vi "Knob.vi"(8 "error in":errorcluster, 11 "Gen Refnum":refnum<vi>) -> (0 "error out":errorcluster, 3 "Knob out":refnum<class "Knob.lvclass">)   [LabVIEW 2014, in "Raspberry Pi Compatible Compiler for LabVIEW.lvlib" / "Knob.lvclass"]
uses:
  Knob.lvclass
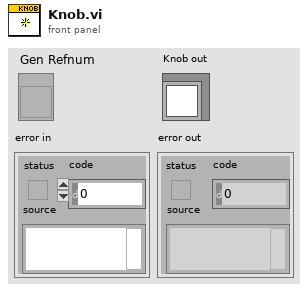
[diagram p1: front panel]
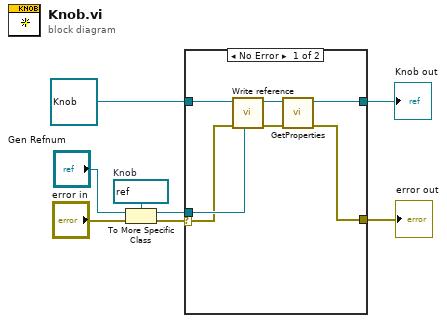
[diagram p0: block diagram]
diagram:
  w2 = refnum<vi> refnum  # Knob
  n1 = To More Specific Class(target class=w2, reference="Gen Refnum", error in="error in") -> (specific class reference=w3:refnum<vi>, error out=w1:errorcluster)
  n2 = case shown="No Error" w1 {
    selector: w1 -> [w13 w16]
    tunnel: refnum<class "Knob.lvclass"> refnum ("Knob in") -> [w15 w17]
    tunnel: [w10 w17] -> w7
    tunnel: [w9 w16] -> w6
    tunnel: w3 -> [w14 _]
    frame No Error {
      n3 = call-dynamic "Write reference.vi"("reference"=w14, "error in"=w13, "GObject in"=w15) -> ("error out"=w12:errorcluster, "GObject out"=w11:refnum<class "Knob.lvclass">)  [unwired: 5 in]
      n4 = call-dynamic "GetProperties.vi"("error in"=w12, "Knob in"=w11) -> ("error out"=w9:errorcluster, "Knob out"=w10:refnum<class "Knob.lvclass">)  [unwired: 8 in]
    }
    frame Error {
    }
  }
  "error out" <- w6
  "Knob out" <- w7
